vi "Twist Drive.vi"   [LabVIEW 2014]
types:
  T1 = cluster{"Buttons":cluster{"1":bool, "2":bool, "3":bool, "4":bool, "5":bool, "6":bool, "7":bool, "8":bool, "9":bool, "10":bool}, "Axes":cluster{"X":dbl, "Y":dbl, "Twist":dbl, "Throttle":dbl}}
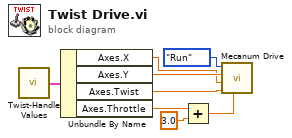
[diagram p0: block diagram]
diagram:
  n1 = call "Twist-Handle Values.vi"() -> ("Twist-Handle"=w8:T1)
  n2 = Unbundle By Name(w8) -> ("Axes.X"=w5:dbl, "Axes.Y"=w6:dbl, "Axes.Twist"=w4:dbl, "Axes.Throttle"=w3:dbl)
  n3 = Add(x=w3, y=3.0) -> (x+y=w1:dbl)
  n4 = call "Mecanum Drive.vi"("Division"=w1, "Turn"=w4, "Strafe"=w5, "Forward/Backward"=w6, "Mode"=enum8{"Start", "Run", "Finish"}."Run") -> ()  [unwired: 7 in]
